vi "Get System Stats.vi"() -> (1 "error out":errorcluster, 2 "Memory info":T1, 3 "CPU Info":T2)   [LabVIEW 2025, in "Simple MCP Server.lvlib"]
doc: "Adds two number x and y."
uses:
  Simple MCP Server.lvlib
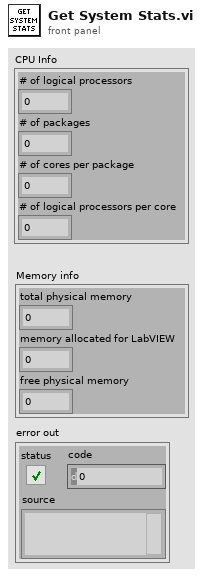
[diagram p1: front panel]
types:
  T1 = cluster{"total physical memory":u64, "memory allocated for LabVIEW":u64, "free physical memory":u64}
  T2 = cluster{"# of logical processors":i32, "# of packages":i32, "# of cores per package":i32, "# of logical processors per core":i32}
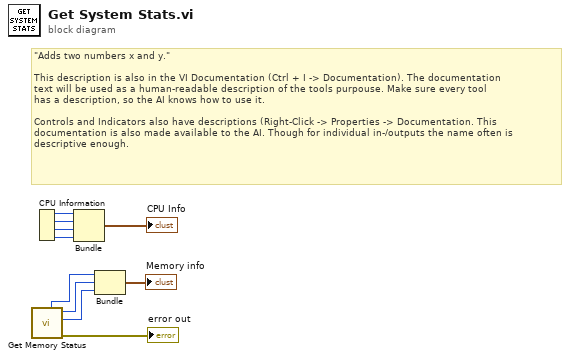
[diagram p0: block diagram]
diagram:
  # "\"Adds two numbers x and y.\"\n\nThis description is also in the VI Documentation (Ctrl + I -> Documentation). The documentation\ntext will be used as a human-readable description of the tools purpouse. Make sure every tool\nhas a description, so the AI knows how to use it.\n\nControls and Indicators also have descriptions (Right-Click -> Properties -> Documentation. This \ndocumentation is also made available to the AI. Though for individual in-/outputs the name often is\ndescriptive enough."
  n1 = CPU Information() -> (4:w10:i32, 5:w9:i32, 6:w8:i32, 7:w7:i32)
  n2 = call <vilib>:"Get Memory Status.vi"() -> ("error out"=→"error out":errorcluster, "free physical memory"=w3:u64, "memory allocated for LabVIEW"=w4:u64, "total physical memory"=w5:u64)  [unwired: 8 in]
  n3 = Bundle("# of logical processors"=w10, "# of packages"=w9, "# of cores per package"=w8, "# of logical processors per core"=w7) -> (→"CPU Info":T2)  [unwired: 1 in]
  n4 = Bundle("total physical memory"=w5, "memory allocated for LabVIEW"=w4, "free physical memory"=w3) -> (→"Memory info":T1)  [unwired: 1 in]
